vi "Digital_Bridge_3_kart.vi"() -> ()   [LabVIEW 2014] (continued)
        frame Enabled {
        }
      }
      n170 = property class="DAQmx Buffer"(reference=w121, error in=w120, "Input:Buffer Size"=w68) -> (reference out=w80:refnum<k21>, error out=w79:errorcluster)
      n171 = property class="DAQmx Buffer"(reference=w116, error in=w117, "Input:Buffer Size"=w68) -> (reference out=w119:refnum<k21>, error out=w118:errorcluster)
      n172 = property class="DAQmx Buffer"(reference=w115, error in=w114, "Input:Buffer Size"=w68) -> (reference out=w113:refnum<k21>, error out=w112:errorcluster)
      n173 = property class="DAQmx Timing"(reference=w80, error in=w79, "More:Reference Clock:Source"=w58, "RefClk.Rate"=w59) -> (reference out=w78:refnum<k21>, error out=w77:errorcluster)
      n174 = call "Get_Terminal_Name_with_Device_Prefix.vi"("error in (no error)"=w77, "Local Terminal Name"="SyncPulse", "task/channels in"=w78) -> ("error out"=w74:errorcluster, "Terminal Name with Device Prefix"=w60:tag, "task out"=w76:refnum<k21>)  [unwired: 6 in]
      n175 = disable-structure shown="Disabled" {
        disable-tunnel: [w527 _] -> w65
        disable-tunnel: [w526 _] -> w64
        disable-tunnel: w62 -> [w525 _]
        disable-tunnel: w61 -> [w524 _]
        disable-tunnel: w60 -> [w523 _]
        disable-tunnel: w59 -> [w522 _]
        disable-tunnel: w58 -> [w521 _]
        frame Disabled {
          n176 = property class="DAQmx Timing"(reference=w525, error in=w524, "More:Reference Clock:Source"=w521, "RefClk.Rate"=w522, "SyncPulse.Src"=w523) -> (reference out=w527:refnum<k21>, error out=w526:errorcluster)
        }
        frame Enabled {
        }
      }
      n177 = disable-structure shown="Disabled" {
        disable-tunnel: w67 -> [w463 _]
        disable-tunnel: w66 -> [w462 _]
        disable-tunnel: w60 -> [w461 _]
        disable-tunnel: w59 -> [w460 _]
        disable-tunnel: w58 -> [w459 _]
        disable-tunnel: [w458 _] -> w54
        disable-tunnel: [w457 _] -> w53
        frame Disabled {
          n178 = property class="DAQmx Timing" props=["More:Reference Clock:Source", "More:Reference Clock:Rate", "SyncPulse.Src", "SyncPulse.SyncTime"](reference=w463, error in=w462, "More:Reference Clock:Source"=w459, "More:Reference Clock:Rate"=w460, "SyncPulse.Src"=w461) -> (reference out=w458:refnum<k21>, error out=w457:errorcluster)  [unwired: 1 out]
        }
        frame Enabled {
        }
      }
      n179 = property class="DAQmx Timing"(reference=w119, error in=w118, "More:Reference Clock:Source"=w58, "More:Reference Clock:Rate"=w59, "SyncPulse.Src"=w60) -> (reference out=w98:refnum<k21>, error out=w97:errorcluster, "SyncPulse.SyncTime"=w72:dbl)
      n180 = property class="DAQmx Timing" props=["More:Reference Clock:Source", "More:Reference Clock:Rate", "SyncPulse.Src", "SyncPulse.SyncTime"](reference=w113, error in=w112, "More:Reference Clock:Source"=w58, "More:Reference Clock:Rate"=w59, "SyncPulse.Src"=w60) -> (reference out=w96:refnum<k21>, error out=w95:errorcluster)  [unwired: 1 out]
      n181 = property class="DAQmx Timing"(reference=w209, error in=w208, "More:Reference Clock:Source"=w58, "RefClk.Rate"=w59, "SyncPulse.Src"=w60) -> (reference out=w92:refnum<k21>, error out=w91:errorcluster)
      n182 = property class="DAQmx Timing"(reference=w149, error in=w148, "More:Reference Clock:Source"=w58, "RefClk.Rate"=w59, "SyncPulse.Src"=w60) -> (reference out=w82:refnum<k21>, error out=w81:errorcluster)
      n183 = property class="DAQmx Timing"(reference=w147, error in=w146, "More:Reference Clock:Source"=w58, "RefClk.Rate"=w59, "SyncPulse.Src"=w60) -> (reference out=w87:refnum<k21>, error out=w88:errorcluster)
      n184 = property class="DAQmx Timing"(reference=w76, error in=w74, "SyncPulse.MinDelayToStart"=w72) -> (reference out=w75:refnum<k21>, error out=w73:errorcluster)
      n185 = call <vilib>:"Basic Function Generator.vi"("sampling info"=w122, "signal type"=w123) -> ("signal out"=w207:waveform(dbl))  [unwired: 7 in, 2 out]
      n186 = call <vilib>:"Basic Function Generator.vi"("sampling info"=w122, "signal type"=w123, "phase"=0.0) -> ("signal out"=w206:waveform(dbl))  [unwired: 6 in, 2 out]
      n187 = Build Array(w207, w206) -> (w57:waveform(dbl)[])
      n188 = call "Get Full Terminal Name.vi"("error in"=w73, "Local Terminal Name"="ai/StartTrigger", "task/channels in"=w75) -> ("error out"=w93:errorcluster, "Terminal Name with Device Prefix"=w63:tag, "task out"=w94:refnum<k21>)  [unwired: 6 in]
      n189 = flat-sequence {
        tunnel: w98 -> [w581]
        tunnel: w97 -> [w580]
        tunnel: w96 -> [w570]
        tunnel: w95 -> [w569]
        tunnel: [w571] -> w43
        tunnel: [w568] -> w44
        tunnel: [w579] -> w48
        tunnel: [w578] -> w46
        tunnel: w94 -> [w577]
        tunnel: [w577] -> w52
        tunnel: [w576] -> w50
        tunnel: w93 -> [w576]
        tunnel: w63 -> [w567]
        tunnel: w54 -> [w575]
        tunnel: w53 -> [w574]
        tunnel: [w573] -> w40
        tunnel: [w572] -> w38
        frame #0 {
          n190 = disable-structure shown="Disabled" {
            disable-tunnel: w575 -> [w586 _]
            disable-tunnel: w574 -> [w585 _]
            disable-tunnel: [w584 _] -> w573
            disable-tunnel: [w583 _] -> w572
            disable-tunnel: w567 -> [w582 _]
            frame Disabled {
              n191 = call-poly <vilib>:"DAQmx Trigger.vi"("task/channels in"=w586, "source"=w582, "error in"=w585) -> ("task out"=w588:refnum<k21>, "error out"=w587:errorcluster)  [unwired: 11 in]
              n192 = call <vilib>:"DAQmx Start Task.vi"("task/channels in"=w588, "error in"=w587) -> ("task out"=w584:refnum<k21>, "error out"=w583:errorcluster)  [unwired: 12 in]
            }
            frame Enabled {
            }
          }
          n193 = call-poly <vilib>:"DAQmx Trigger.vi"("task/channels in"=w581, "source"=w567, "error in"=w580) -> ("task out"=w579:refnum<k21>, "error out"=w578:errorcluster)  [unwired: 11 in]
          n194 = call-poly <vilib>:"DAQmx Trigger.vi"("task/channels in"=w570, "source"=w567, "error in"=w569) -> ("task out"=w571:refnum<k21>, "error out"=w568:errorcluster)  [unwired: 11 in]
        }
      }
      n195 = disable-structure shown="Disabled" {
        disable-tunnel: w65 -> [w514 _]
        disable-tunnel: w64 -> [w513 _]
        disable-tunnel: w63 -> [w512 _]
        disable-tunnel: w57 -> [w511 _]
        disable-tunnel: [w510 _] -> w56
        disable-tunnel: [w509 _] -> w55
        frame Disabled {
          w518 = 10.0  # timeout (s)
          w517 = FALSE  # auto start
          n196 = call-poly <vilib>:"DAQmx Trigger.vi"("task/channels in"=w514, "source"=w512, "error in"=w513) -> ("task out"=w519:refnum<k21>, "error out"=w520:errorcluster)  [unwired: 11 in]
          n197 = call-poly <vilib>:"DAQmx Write.vi"("task/channels in"=w519, "auto start"=w517, "data"=w511, "timeout"=w518, "error in"=w520) -> ("task out"=w516:refnum<k21>, "error out"=w515:errorcluster)  [unwired: 8 in, 1 out]
          n198 = call <vilib>:"DAQmx Start Task.vi"("task/channels in"=w516, "error in"=w515) -> ("task out"=w510:refnum<k21>, "error out"=w509:errorcluster)  [unwired: 12 in]
        }
        frame Enabled {
        }
      }
      n199 = call-poly <vilib>:"DAQmx Trigger.vi"("task/channels in"=w87, "source"=w63, "error in"=w88) -> ("task out"=w86:refnum<k21>, "error out"=w85:errorcluster)  [unwired: 11 in]
      n200 = call-poly <vilib>:"DAQmx Trigger.vi"("task/channels in"=w92, "source"=w63, "error in"=w91) -> ("task out"=w90:refnum<k21>, "error out"=w89:errorcluster)  [unwired: 11 in]
      n201 = call-poly <vilib>:"DAQmx Trigger.vi"("task/channels in"=w82, "source"=w63, "error in"=w81) -> ("task out"=w83:refnum<k21>, "error out"=w84:errorcluster)  [unwired: 11 in]
      n202 = flat-sequence {
        tunnel: w52 -> [w566]
        tunnel: [w566] -> w51
        tunnel: w50 -> [w565]
        tunnel: [w565] -> w49
        tunnel: w48 -> [w564]
        tunnel: [w564] -> w47
        tunnel: w46 -> [w563]
        tunnel: [w563] -> w45
        tunnel: w44 -> [w562]
        tunnel: w43 -> [w561]
        tunnel: [w560] -> w42
        tunnel: [w559] -> w41
        tunnel: w40 -> [w558]
        tunnel: [w558] -> w39
        tunnel: w38 -> [w557]
        tunnel: [w557] -> w37
        frame #0 {
          n203 = call <vilib>:"DAQmx Start Task.vi"("task/channels in"=w561, "error in"=w562) -> ("task out"=w560:refnum<k21>, "error out"=w559:errorcluster)  [unwired: 12 in]
        }
      }
      n204 = call-poly <vilib>:"DAQmx Write.vi"("task/channels in"=w83, "auto start"=w139, "data"=w57, "timeout"=w138, "error in"=w84) -> ("task out"=w140:refnum<k21>, "error out"=w141:errorcluster)  [unwired: 8 in, 1 out]
      n205 = call-poly <vilib>:"DAQmx Write.vi"("task/channels in"=w86, "auto start"=w144, "data"=w57, "timeout"=w145, "error in"=w85) -> ("task out"=w143:refnum<k21>, "error out"=w142:errorcluster)  [unwired: 8 in, 1 out]
      n206 = call-poly <vilib>:"DAQmx Write.vi"("task/channels in"=w90, "auto start"=w211, "data"=w57, "timeout"=w210, "error in"=w89) -> ("task out"=w214:refnum<k21>, "error out"=w215:errorcluster)  [unwired: 8 in, 1 out]
      n207 = call <vilib>:"DAQmx Start Task.vi"("task/channels in"=w47, "error in"=w45) -> ("task out"=w351:refnum<k21>, "error out"=w350:errorcluster)  [unwired: 12 in]
      n208 = call <vilib>:"DAQmx Start Task.vi"("task/channels in"=w140, "error in"=w141) -> ("task out"=w131:refnum<k21>, "error out"=w130:errorcluster)  [unwired: 12 in]
      n209 = call <vilib>:"DAQmx Start Task.vi"("task/channels in"=w143, "error in"=w142) -> ("task out"=w136:refnum<k21>, "error out"=w137:errorcluster)  [unwired: 12 in]
      n210 = call <vilib>:"DAQmx Start Task.vi"("task/channels in"=w214, "error in"=w215) -> ("task out"=w212:refnum<k21>, "error out"=w213:errorcluster)  [unwired: 12 in]
      n211 = flat-sequence {
        tunnel: w351 -> [w6985]
        tunnel: w350 -> [w6984]
        tunnel: [w6985] -> w347
        tunnel: [w6984] -> w346
        tunnel: [w6983] -> w348
        tunnel: [w6982] -> w349
        tunnel: w51 -> [w6981]
        tunnel: w49 -> [w6980]
        frame #0 {
          n212 = call <vilib>:"DAQmx Start Task.vi"("task/channels in"=w6981, "error in"=w6980) -> ("task out"=w6982:refnum<k21>, "error out"=w6983:errorcluster)  [unwired: 12 in]
        }
      }
      n213 = while {
        stop <- w352 stop-if-true
        n214 = event shown="[3] \"Manuel Setup\": Mouse Down" {
          selector: _ -> [_ _ _ _ _ _]
          dyn-events: _ -> [_ _ _ _ _ _]
          timeout: _ -> [_ _ _ _ _ _]
          event Timeout {
            n215 = event-data() -> ()  [unwired: 1 in, 3 out]
            n216 = flat-sequence {
              frame #0 {
              }
            }
          }
          event "Frekans Listbox": Double Click {
            n217 = event-data() -> ("Row"=w354:i32)  [unwired: 1 in, 8 out]
            n218 = flat-sequence {
              tunnel: w354 -> [w355]
              frame #0 {
                n219 = property on="Frekans Listbox" class="LstBox (strict)"() -> ("Item Symbols"=w359:i32[])  [unwired: 2 in, 2 out]
                n220 = Index Array(array=w359, index=w355) -> (element=w358:i32)
                n221 = Equal?(x=w358, y=10) -> (x = y?=w356:bool)
                n222 = case shown="True" w356 {
                  tunnel: w355 -> [w360 w364]
                  frame False {
                    n223 = property on="Frekans Listbox" class="LstBox (strict)"() -> ("Item Symbols"=w363:i32[])  [unwired: 2 in, 2 out]
                    n224 = Replace Array Subset(array=w363, new element=10 ("new element/subarray"), index=w360) -> (w362:i32[])
                    n225 = property on="Frekans Listbox" class="LstBox (strict)"("Item Symbols"=w362) -> ()  [unwired: 2 in, 2 out]
                  }
                  frame True {
                    n226 = property on="Frekans Listbox" class="LstBox (strict)"() -> ("Item Symbols"=w367:i32[])  [unwired: 2 in, 2 out]
                    n227 = Replace Array Subset(array=w367, new element=1 ("new element/subarray"), index=w364) -> (w366:i32[])
                    n228 = property on="Frekans Listbox" class="LstBox (strict)"("Item Symbols"=w366) -> ()  [unwired: 2 in, 2 out]
                  }
                }
              }
            }
          }
          event "Default Values Listbox": Double Click {
            n229 = event-data() -> ("Row"=w370:i32)  [unwired: 1 in, 8 out]
            n230 = flat-sequence {
              tunnel: w370 -> [w371]
              tunnel: [w372] -> w369
              tunnel: [w371] -> w368
              tunnel: w369 -> [w377]
              tunnel: w368 -> [w376]
              frame #0 {
                n231 = property on="Default Values Listbox" class="LstBox (strict)"() -> ("Item Symbols"=w375:i32[])  [unwired: 2 in, 2 out]
                n232 = Index Array(array=w375, index=w371) -> (element=w374:i32)
                n233 = Equal?(x=w374, y=10) -> (x = y?=w372:bool)
              }
              frame #1 {
                n234 = case shown="True" w377 {
                  tunnel: w376 -> [w378 w402]
                  frame False {
                    n235 = flat-sequence {
                      tunnel: [w382] -> w381
                      tunnel: w378 -> [w382]
                      tunnel: [w382] -> w380
                      tunnel: w381 -> [w390]
                      tunnel: [w387] -> w379
                      tunnel: w380 -> [w387]
                      tunnel: w379 -> [w391]
                      frame #0 {
                      }
                      frame #1 {
                        n236 = local read "F Values Array"() -> (w383:dbl[][])
                        n237 = control-ref of="Default Values Listbox"() -> (w384:refnum<vi>)
                        n238 = property on="Default Values Listbox" class="LstBox (strict)"() -> ("Item Names"=w389:string[])  [unwired: 2 in, 2 out]
                        n239 = Fract/Exp String To Number(string=w389) -> (number=w388:dbl[])  [unwired: 3 in, 1 out]
                        n240 = Index Array(array=w388, index=w390) -> (element=w386:dbl)
                        n241 = call "delete_values.vi"("F values array"=w383, "Frekans"=w386, "LstBox Refnum"=w384) -> ("Output F values array"=w385:dbl[][])  [unwired: 8 in]
                        n242 = local write "F Values Array"(w385) -> ()
                      }
                      frame #2 {
                        n243 = property on="Default Values Listbox" class="LstBox (strict)"() -> ("Item Symbols"=w394:i32[])  [unwired: 2 in, 2 out]
                        n244 = Replace Array Subset(array=w394, new element=10 ("new element/subarray"), index=w391) -> (w393:i32[])
                        n245 = property on="Default Values Listbox" class="LstBox (strict)"("Item Symbols"=w393) -> ()  [unwired: 2 in, 2 out]
                      }
                    }
                  }
                  frame True {
                    n246 = flat-sequence {
                      tunnel: [w405] -> w403
                      tunnel: w402 -> [w405]
                      tunnel: [w406] -> w401
                      tunnel: [w405] -> w400
                      tunnel: w403 -> [w408]
                      tunnel: w401 -> [w415]
                      tunnel: [w412] -> w398
                      tunnel: w400 -> [w412]
                      tunnel: [w408] -> w396
                      tunnel: w398 -> [w420]
                      tunnel: [w420] -> w397
                      tunnel: w396 -> [w419]
                      tunnel: [w419] -> w395
                      tunnel: w397 -> [w423]
                      tunnel: [w423] -> w399
                      tunnel: w395 -> [w421]
                      tunnel: w399 -> [w424]
                      frame #0 {
                        n247 = local read "Sheet name"() -> (w404:string)
                        n248 = call "Excel Get Data Specified Field.vi"("SheetName"=w404) -> ("data"=w407:string[][])  [unwired: 4 in, 2 out]
                        n249 = Fract/Exp String To Number(string=w407) -> (number=w406:dbl[][])  [unwired: 3 in, 1 out]
                      }
                      frame #1 {
                        n250 = local read "F Values Array"() -> (w409:dbl[][])
                        n251 = control-ref of="Default Values Listbox"() -> (w410:refnum<vi>)
                        n252 = Reshape Array(w415, 51 ("dimension size")) -> (w413:dbl[])
                        n253 = property on="Default Values Listbox" class="LstBox (strict)"() -> ("Item Names"=w418:string[])  [unwired: 2 in, 2 out]
                        n254 = Fract/Exp String To Number(string=w418) -> (number=w417:dbl[])  [unwired: 3 in, 1 out]
                        n255 = Index Array(array=w417, index=w408) -> (element=w416:dbl)
                        n256 = call "add_values.vi"("F values array"=w409, "Values"=w413, "Frekans"=w416, "LstBox Refnum"=w410) -> ("Output F values array"=w411:dbl[][])  [unwired: 7 in]
                        n257 = local write "F Values Array"(w411) -> ()
                      }
                      frame #2 {
                      }
                      frame #3 {
                        n258 = local read "F Values Array"() -> (w422:dbl[][])
                        n259 = call "rlc warning.vi"("frekans index"=w421, "F values array"=w422) -> ()  [unwired: 10 in]
                      }
                      frame #4 {
                        n260 = property on="Default Values Listbox" class="LstBox (strict)"() -> ("Item Symbols"=w427:i32[])  [unwired: 2 in, 2 out]
                        n261 = Replace Array Subset(array=w427, new element=1 ("new element/subarray"), index=w424) -> (w426:i32[])
                        n262 = property on="Default Values Listbox" class="LstBox (strict)"("Item Symbols"=w426) -> ()  [unwired: 2 in, 2 out]
                      }
                    }
                  }
                }
              }
            }
          }
          event "Manuel Setup": Mouse Down {
            n263 = event-data() -> ()  [unwired: 1 in, 8 out]
            n264 = local read "Sheet name"() -> (w431:string)
            n265 = call "Excel Get Data Specified Field.vi"("SheetName"=w431) -> ("data"=w432:string[][])  [unwired: 4 in, 2 out]
            n266 = Fract/Exp String To Number(string=w432) -> (number=w433:dbl[][])  [unwired: 3 in, 1 out]
            n267 = Reshape Array(w433, 51 ("dimension size")) -> (w428:dbl[])
            n268 = for {
              N: 51 -> [_]
              tunnel: w428 -> [w435]
              i -> [w436]
              n269 = Index Array(array=w435, index=w436) -> (element=w434:dbl)
              n270 = case shown="0, Default" w436 {
                tunnel: w434 -> [w437 w438 _ _ _ _ _ _ _ w439 w440 w441 w442 w443 _ _ _ _ _ w444 w445 w446 w447 w448 _ _ _ _ _ _ _ _ _ _ _ _ _ _ _ _ _ _ _ _ _ _ _ _ _ _ _]
                frame 0, Default {
                  n271 = global write "DB_Global_4_kart-Test.vi" "Frequency"(w437) -> ()
                }
                frame 1 {
                  n272 = global write "DB_Global_4_kart-Test.vi" "amplitude 1/0"(w438) -> ()
                }
                frame 2 {
                }
                frame 3 {
                }
                frame 4 {
                }
                frame 5 {
                }
                frame 6 {
                }
                frame 7 {
                }
                frame 8 {
                }
                frame 9 {
                  n273 = global write "DB_Global_4_kart-Test.vi" "amplitude 2/0"(w439) -> ()
                }
                frame 10 {
                  n274 = global write "DB_Global_4_kart-Test.vi" "amplitude 3/0"(w440) -> ()
                }
                frame 11 {
                  n275 = global write "DB_Global_4_kart-Test.vi" "amplitude 3/1"(w441) -> ()
                }
                frame 12 {
                  n276 = global write "DB_Global_4_kart-Test.vi" "amplitude 1/1"(w442) -> ()
                }
                frame 13 {
                  n277 = global write "DB_Global_4_kart-Test.vi" "amplitude 2/1"(w443) -> ()
                }
                frame 14 {
                }
                frame 15 {
                }
                frame 16 {
                }
                frame 17 {
                }
                frame 18 {
                }
                frame 19 {
                  n278 = global write "DB_Global_4_kart-Test.vi" "phase 2/ 0"(w444) -> ()
                }
                frame 20 {
                  n279 = global write "DB_Global_4_kart-Test.vi" "phase 3/0"(w445) -> ()
                }
                frame 21 {
                  n280 = global write "DB_Global_4_kart-Test.vi" "phase 3/1"(w446) -> ()
                }
                frame 22 {
                  n281 = global write "DB_Global_4_kart-Test.vi" "phase 1/1"(w447) -> ()
                }
                frame 23 {
                  n282 = global write "DB_Global_4_kart-Test.vi" "phase 2/1"(w448) -> ()
                }
                frame 24 {
                }
                frame 25 {
                }
                frame 26 {
                }
                frame 27 {
                }
                frame 28 {
                }
                frame 29 {
                }
                frame 30 {
                }
                frame 31 {
                }
                frame 32 {
                }
                frame 33 {
                }
                frame 34 {
                }
                frame 35 {
                }
                frame 36 {
                }
                frame 37 {
                }
                frame 38 {
                }
                frame 39 {
                }
                frame 40 {
                }
                frame 41 {
                }
                frame 42 {
                }
                frame 43 {
                }
                frame 44 {
                }
                frame 45 {
                }
                frame 46 {
                }
                frame 47 {
                }
                frame 48 {
                }
                frame 49 {
                }
                frame 50 {
                }
              }
            }
          }
          event "Multicolumn Listbox": Mouse Down {
            n283 = event-data() -> ("Coords"=w450:T8)  [unwired: 1 in, 7 out]
            n284 = invoke on="Multicolumn Listbox" class="MCListbox (strict)" method="Point To Row Column"("Point"=w450) -> ("CellPosition"=w449:T9)  [unwired: 6 in, 6 out]
            n285 = property on="Multicolumn Listbox" class="MCListbox (strict)"("EditPos"=w449) -> ()  [unwired: 2 in, 2 out]
          }
          event "Manuel Input": Mouse Down {
            n286 = event-data() -> ()  [unwired: 1 in, 8 out]
            n287 = call <vilib>:"System Exec.vi"("command line"="cmd /c start \"\" \"D:\\Projeler\\Digital Bridge\\Digital_Bridge_3_kart\\Manuel.vi\"") -> ()  [unwired: 7 in, 4 out]
          }
        }
        n288 = Wait (ms)(milliseconds to wait=u32 50) -> ()  [unwired: 1 out]
        n289 = local read "stop listbox"() -> (w352:bool)
      }
      n290 = while {
        shift-right: [w636] -> w344
        shift-left: w348 -> [w636]
        shift-right: [w634] -> w340
        shift-left: w346 -> [w634]
        shift-right: [w637] -> w345
        shift-left: w349 -> [w637]
        shift-right: [w635] -> w341
        shift-left: w347 -> [w635]
        shift-right: [w633] -> w332
        shift-left: w42 -> [w633]
        shift-right: [w632] -> w331
        shift-left: w41 -> [w632]
        shift-right: [w640] -> w203
        shift-left: w213 -> [w655]
        shift-right: [w654] -> w204
        shift-left: w212 -> [w653]
        shift-right: [w639] -> w133
        shift-left: w137 -> [w649]
        shift-right: [w650] -> w132
        shift-left: w136 -> [w651]
        shift-right: [w645] -> w127
        shift-left: w131 -> [w646]
        shift-right: [w638] -> w126
        shift-left: w130 -> [w644]
        shift-right: [w627] -> w36
        shift-left: w56 -> [w629]
        shift-right: [w626] -> w35
        shift-left: w55 -> [w628]
        shift-right: [w625] -> w33
        shift-left: w39 -> [w625]
        shift-right: [w624] -> w32
        shift-left: w37 -> [w624]
        stop <- w619 stop-if-true
        w652 = FALSE  # auto start
        # "Bu bölümde, input değerleri sürekli güncellenir. \n\nGüncel tutulan bu input değerleri, daha sonra Excel dosyasına aktarılacak ölçüm sonuçlarıdır."
        # "Bu bölümde, denge koşullarını değiştirmek istediğimiz listbox’un kodları bulunur. \n\nYani, kullanıcının listbox üzerinden seçtiği denge koşullarına göre programın davranışını belirleyen işlemler burada gerçekleştirilir."
        # "Bu bölüm, eğer giriş değeri 8V’dan büyükse ya da ölçüm sayısı (meas number) belirlenen sınırı aşarsa aktif olur. \n\nBu durumda, ilgili frekans için “dengelenemedi” mesajı atanır. \n\nAncak program, sonraki turlarda bu frekans için tekrar dengeleme denemelerine devam eder."
        # "Bu bölüm, ya tüm dengeler başarıyla sağlandığında ya da bir hata (error) durumunda aktif olur. \n\nEğer ölçüm yapılan frekansta dengeleme tamamlanmışsa, program mevcut frekanstan doğrudan sonraki frekansa geçiş yapar. \n\nHata oluşmuşsa da yine diğer frekansa geçiş için gerekli hazırlıklar burada yapılır. \n\nKısaca, bu case bir frekans tamamlandığında diğerine geçiş için ön hazırlıkların yapıldığı yerdir."
        # "Bu bölüm, program ilk kez başlatıldığında yapılması gereken başlangıç işlemlerini içerir. \n\nÖrneğin; faz için 2 boyutlu dizilerin (2D array) oluşturulması, programdaki birçok değişkenin ve değerlerin sıfırlanması gibi temel ayarlamalar burada yapılır. \n\nBu sayede program, temiz ve hazır bir durumda çalışmaya başlar."
        # "BASLAT: \n\nBu bölüm, kullanıcı ana programda gerekli tüm ayarları yaptıktan sonra \"Başlat\" düğmesine bastığında çalışır. Programın başlamasından önce bazı kontroller yapılır. Örneğin, kullanıcı geçerli bir frekans seçmiş mi, ölçüm ve set değerleri 100’ün üzerinde mi, gerekli global giriş değerleri girilmiş mi gibi durumlar kontrol edilir. Bu kontroller sayesinde eksik veya hatalı girişler varsa kullanıcıya uyarı verilir. \n\nAynı zamanda bu bölüm, programın düzgün çalışabilmesi için gerekli olan temel verilerin oluşturulduğu alandır. Control Hz, frekanslar, ekstra varsayılan değerler, denge fazlarını içeren diziler ve bazı cluster yapıları burada tanımlanır. Eğer kullanıcı Excel’den veri aldıysa, bu veriler de burada işlenerek F values dizisine aktarılır. Kısacası, programın başlaması için gerekli olan tüm başlangıç ayarları ve veri hazırlıkları bu case içinde yapılır."
        # "Dev3"
        # "Dev2"
        # "Dev1"
        # "Slot2"
        n291 = flat-sequence {
          tunnel: [w4175] -> w601
          tunnel: [w4174] -> w600
          tunnel: [w4173] -> w599
          tunnel: [w4179] -> w621
          tunnel: w601 -> [w4180]
          tunnel: w600 -> [w4181]
          tunnel: w599 -> [w4178]
          tunnel: [w4245] -> w643
          tunnel: [w4237] -> w642
          tunnel: [w4234] -> w641
          tunnel: [w4193] -> w630
          tunnel: w621 -> [w4189]
          frame #0 {
            n292 = local read "frekans index"() -> (w4176:dbl)
            n293 = local read "Frekanslar"() -> (w4177:dbl[])
            n294 = global read "DB_Global_4_kart-Test.vi" "Manuel Kullan"() -> (w4174:bool)
            n295 = global read "DB_Global_4_kart-Test.vi" "Frequency"() -> (w4175:dbl)
            n296 = Index Array(array=w4177, index=w4176) -> (element=w4173:dbl)
          }
          frame #1 {
            n297 = case shown="False" w4181 {
              tunnel: [w4183 w4188] -> w4179
              tunnel: w4180 -> [_ w4188]
              tunnel: w4178 -> [w4182 _]
              frame False {
                n298 = Less Or Equal?(x=w4182, y=0.0) -> (x <= y?=w4184:bool)
                n299 = case shown="True" w4184 {
                  tunnel: [w4186 1000.0] -> w4183
                  tunnel: w4182 -> [w4186 _]
                  frame False {
                  }
                  frame True {
                  }
                }
              }
              frame True {
              }
            }
          }
          frame #2 {
            w4192 = 0.0 ("Offset")
            # "Yedek Kart ao1"
            # "Yedek Kart ao0"
            # "1R Voltajı"
            # "Kelvin Voltajı"
            # "Wagner Voltajı"
            # "10R Voltajı"
            # "Ana Denge Voltajı"
            # "Besleme Voltajı"
            n300 = global read "DB_Global_4_kart-Test.vi" "amplitude 1/0"() -> (w4214:dbl)
            n301 = global read "DB_Global_4_kart-Test.vi" "phase 1/ 0"() -> (w4212:dbl)
            n302 = global read "DB_Global_4_kart-Test.vi" "amplitude 1/1"() -> (w4213:dbl)
            n303 = global read "DB_Global_4_kart-Test.vi" "phase 1/1"() -> (w4218:dbl)
            n304 = global read "DB_Global_4_kart-Test.vi" "amplitude 2/0"() -> (w4232:dbl)
            n305 = global read "DB_Global_4_kart-Test.vi" "phase 2/ 0"() -> (w4233:dbl)
            n306 = global read "DB_Global_4_kart-Test.vi" "amplitude 2/1"() -> (w4211:dbl)
            n307 = global read "DB_Global_4_kart-Test.vi" "phase 2/1"() -> (w4210:dbl)
            n308 = global read "DB_Global_4_kart-Test.vi" "amplitude 3/0"() -> (w4228:dbl)
            n309 = global read "DB_Global_4_kart-Test.vi" "phase 3/0"() -> (w4227:dbl)
            n310 = global read "DB_Global_4_kart-Test.vi" "amplitude 3/1"() -> (w4223:dbl)
            n311 = global read "DB_Global_4_kart-Test.vi" "phase 3/1"() -> (w4222:dbl)
            n312 = global read "DB_Global_4_kart-Test.vi" "amplitude 5/0"() -> (w4199:dbl)
            n313 = global read "DB_Global_4_kart-Test.vi" "phase 5/0"() -> (w4198:dbl)
            n314 = global read "DB_Global_4_kart-Test.vi" "amplitude 5/1"() -> (w4202:dbl)
            n315 = global read "DB_Global_4_kart-Test.vi" "phase 5/1"() -> (w4203:dbl)
            n316 = global write "DB_Global_4_kart-Test.vi" "Frequency"(w4189) -> ()
            n317 = Re/Im To Polar(2:w4203, 3:w4202) -> (0:w4205:dbl, 1:w4204:dbl)
            n318 = Re/Im To Polar(2:w4210, 3:w4211) -> (0:w4208:dbl, 1:w4209:dbl)
            n319 = Re/Im To Polar(2:w4198, 3:w4199) -> (0:w4200:dbl, 1:w4191:dbl)
            n320 = Re/Im To Polar(2:w4227, 3:w4228) -> (0:w4225:dbl, 1:w4226:dbl)
            n321 = Re/Im To Polar(2:w4222, 3:w4223) -> (0:w4220:dbl, 1:w4221:dbl)
            n322 = Re/Im To Polar(2:w4218, 3:w4213) -> (0:w4216:dbl, 1:w4217:dbl)
            n323 = expression code="(x/pi)*180.0" ("radians to degrees")(w4205) -> (w4206:dbl)
            n324 = expression code="(x/pi)*180.0" ("radians to degrees")(w4208) -> (w4207:dbl)
            n325 = expression code="(x/pi)*180.0" ("radians to degrees")(w4200) -> (w4201:dbl)
            n326 = Re/Im To Polar(2:w4233, 3:w4232) -> (0:w4230:dbl, 1:w4231:dbl)
            n327 = expression code="(x/pi)*180.0" "radians to degrees"(w4220) -> (w4219:dbl)
            n328 = expression code="(x/pi)*180.0" ("radians to degrees")(w4225) -> (w4224:dbl)
            n329 = expression code="(x/pi)*180.0" ("radians to degrees")(w4216) -> (w4215:dbl)
            n330 = expression code="(x/pi)*180.0" ("radians to degrees")(w4230) -> (w4229:dbl)
            n331 = call "Simulate Signal2"("Offset"=w4192, "Reset Signal"=TRUE, "Frequency"=w4189, "Amplitude"=w4217, "Phase"=w4215) -> ("Sine"=w4246:dynamicdata)  [unwired: 9 in, 1 out]
            n332 = call "Simulate Signal8"("Offset"="Yedek Kart offset", "Reset Signal"=TRUE, "Frequency"=w4189, "Amplitude"=w4204, "Phase"=w4206) -> ("Sine"=w4196:dynamicdata)  [unwired: 9 in, 1 out]
            n333 = call "Simulate Signal"("Offset"=w4192, "Reset Signal"=TRUE, "Frequency"=w4189, "Amplitude"=w4214, "Phase"=w4212) -> ("Sine"=w4247:dynamicdata)  [unwired: 9 in, 1 out]
            n334 = call "Simulate Signal7"("Offset"="Yedek Kart offset", "Reset Signal"=TRUE, "Frequency"=w4189, "Amplitude"=w4191, "Phase"=w4201) -> ("Sine"=w4197:dynamicdata)  [unwired: 9 in, 1 out]
            n335 = call "Simulate Signal5"("Offset"=w4192, "Reset Signal"=TRUE, "Frequency"=w4189, "Amplitude"=w4226, "Phase"=w4224) -> ("Sine"=w4235:dynamicdata)  [unwired: 9 in, 1 out]
            n336 = call "Simulate Signal6"("Offset"=w4192, "Reset Signal"=TRUE, "Frequency"=w4189, "Amplitude"=w4221, "Phase"=w4219) -> ("Sine"=w4236:dynamicdata)  [unwired: 9 in, 1 out]
            n337 = call "Simulate Signal3"("Offset"=w4192, "Reset Signal"=TRUE, "Frequency"=w4189, "Amplitude"=w4231, "Phase"=w4229) -> ("Sine"=w4238:dynamicdata)  [unwired: 9 in, 1 out]
            n338 = call "Simulate Signal4"("Offset"=w4192, "Reset Signal"=TRUE, "Frequency"=w4189, "Amplitude"=w4209, "Phase"=w4207) -> ("Sine"=w4239:dynamicdata)  [unwired: 9 in, 1 out]
            n339 = Build Array(w4197, w4196) -> (w4193:dynamicdata[])
            n340 = Build Array(w4235, w4236) -> (w4234:dynamicdata[])
            n341 = Build Array(w4247, w4246) -> (w4245:dynamicdata[])
            n342 = Build Array(w4238, w4239) -> (w4237:dynamicdata[])
          }
        }
        n343 = case shown="True" "BASLAT" {
          tunnel: "Fazları ve ilk denge koşulu dengelemek için gerekli range ve input değerleri verdiniz mi?\n[Bu kısım önemli çünkü ilk range ve input değerleri fazların doğru girilmesi için önem arz ediyor.]" -> [_ w1132]
          frame False {
          }
          frame True {
            n344 = local read "start time"() -> (w1134:string)
            n345 = String Length(string=w1134) -> (length=w1135:i32)
            n346 = Equal?(x=w1135, y=0) -> (x = y?=w1133:bool)
            n347 = case shown="True" w1133 {
              tunnel: [TRUE ("T button?") w1142] -> w1137
              tunnel: w1132 -> [_ w1139]
              frame False {
              }
              frame True {
                n348 = Two Button Dialog(message=w1139, 1:"Ayarla", 2:"Evet") -> (T button?=w1142:bool)
              }
            }
            n349 = case shown="True" w1137 {
              frame False {
                n350 = One Button Dialog(message="Değerleri girdikten sonra ana programı tekrardan başlatmayı unutmayın", button name ("OK")="Tamam") -> (true=w1143:bool)
                n351 = case shown="True" w1143 {
                  frame False {
                  }
                  frame True {
                    n352 = local write "BASLAT"(FALSE ("BASLAT")) -> ()
                    n353 = local write "Stop"(TRUE ("BASLAT")) -> ()
                    n354 = call <vilib>:"System Exec.vi"("command line"="cmd /c start \"\" \"D:\\Projeler\\Digital Bridge\\Digital_Bridge_3_kart\\First_input_values.vi\"") -> ()  [unwired: 7 in, 4 out]
                  }
                }
              }
              frame True {
                n355 = local read "start time"() -> (w1153:string)
                n356 = String Length(string=w1153) -> (length=w1152:i32)
                n357 = Equal?(x=w1152, y=0) -> (x = y?=w1151:bool)
                n358 = case shown="True" w1151 {
                  tunnel: [TRUE w1155] -> w1150
                  frame False {
                  }
                  frame True {
                    n359 = flat-sequence {
                      tunnel: [w1156] -> w1155
                      frame #0 {
                        n360 = control-ref of="Frekans Listbox"() -> (w1160:refnum<vi>)
                        n361 = case shown="0, Default" "Direnc 1 - Direnc 2" {
                          frame 0, Default {
                            n362 = local write "Direnc 1 [ohm]"(1000000.0 ("Direnc 1 [ohm]")) -> ()
                            n363 = local write "Direnc 2 [ohm]"(100000.0 ("Direnc 1 [ohm]")) -> ()
                          }
                          frame 1 {
                            n364 = local write "Direnc 1 [ohm]"(100000.0 ("Direnc 1 [ohm]")) -> ()
                            n365 = local write "Direnc 2 [ohm]"(10000.0 ("Direnc 1 [ohm]")) -> ()
                          }
                          frame 2 {
                            n366 = local write "Direnc 1 [ohm]"(10000.0 ("Direnc 1 [ohm]")) -> ()
                            n367 = local write "Direnc 2 [ohm]"(1000.0 ("Direnc 1 [ohm]")) -> ()
                          }
                          frame 3 {
                            n368 = local write "Direnc 1 [ohm]"(1000.0 ("Direnc 1 [ohm]")) -> ()
                            n369 = local write "Direnc 2 [ohm]"(100.0 ("Direnc 1 [ohm]")) -> ()
                          }
                          frame 4 {
                            n370 = local write "Direnc 1 [ohm]"(100.0 ("Direnc 1 [ohm]")) -> ()
                            n371 = local write "Direnc 2 [ohm]"(10.0 ("Direnc 1 [ohm]")) -> ()
                          }
                          frame 5 {
                            n372 = local write "Direnc 1 [ohm]"(10.0 ("Direnc 1 [ohm]")) -> ()
                            n373 = local write "Direnc 2 [ohm]"(1.0 ("Direnc 1 [ohm]")) -> ()
                          }
                          frame 6 {
                            n374 = local write "Direnc 1 [ohm]"(1000000.0 ("Direnc 1 [ohm]")) -> ()
                            n375 = local write "Direnc 2 [ohm]"(1000000.0 ("Direnc 1 [ohm]")) -> ()
                          }
                          frame 7 {
                            n376 = local write "Direnc 1 [ohm]"(100000.0 ("Direnc 1 [ohm]")) -> ()
                            n377 = local write "Direnc 2 [ohm]"(100000.0 ("Direnc 1 [ohm]")) -> ()
                          }
                          frame 8 {
                            n378 = local write "Direnc 1 [ohm]"(10000.0 ("Direnc 1 [ohm]")) -> ()
                            n379 = local write "Direnc 2 [ohm]"(10000.0 ("Direnc 1 [ohm]")) -> ()
                          }
                          frame 9 {
                            n380 = local write "Direnc 1 [ohm]"(1000.0 ("Direnc 1 [ohm]")) -> ()
                            n381 = local write "Direnc 2 [ohm]"(1000.0 ("Direnc 1 [ohm]")) -> ()
                          }
                          frame 10 {
                            n382 = local write "Direnc 1 [ohm]"(100.0 ("Direnc 1 [ohm]")) -> ()
                            n383 = local write "Direnc 2 [ohm]"(100.0 ("Direnc 1 [ohm]")) -> ()
                          }
                          frame 11 {
                            n384 = local write "Direnc 1 [ohm]"(10.0 ("Direnc 1 [ohm]")) -> ()
                            n385 = local write "Direnc 2 [ohm]"(10.0 ("Direnc 1 [ohm]")) -> ()
                          }
                          frame 12 {
                            n386 = local write "Direnc 1 [ohm]"(1.0 ("Direnc 1 [ohm]")) -> ()
                            n387 = local write "Direnc 2 [ohm]"(1.0 ("Direnc 1 [ohm]")) -> ()
                          }
                          frame 13 {
                            n388 = local write "Direnc 1 [ohm]"(1e-06 ("Direnc 1 [ohm]")) -> ()
                            n389 = local write "Direnc 2 [ohm]"(1e-07 ("Direnc 1 [ohm]")) -> ()
                          }
                          frame 14 {
                            n390 = local write "Direnc 1 [ohm]"(1e-07 ("Direnc 1 [ohm]")) -> ()
                            n391 = local write "Direnc 2 [ohm]"(1e-08 ("Direnc 1 [ohm]")) -> ()
                          }
                          frame 15 {
                            n392 = local write "Direnc 1 [ohm]"(1e-08 ("Direnc 1 [ohm]")) -> ()
                            n393 = local write "Direnc 2 [ohm]"(1e-09 ("Direnc 1 [ohm]")) -> ()
                          }
                          frame 16 {
                            n394 = local write "Direnc 1 [ohm]"(1e-09 ("Direnc 1 [ohm]")) -> ()
                            n395 = local write "Direnc 2 [ohm]"(1e-10 ("Direnc 1 [ohm]")) -> ()
                          }
                          frame 17 {
                            n396 = local write "Direnc 1 [ohm]"(1e-10 ("Direnc 1 [ohm]")) -> ()
                            n397 = local write "Direnc 2 [ohm]"(1e-11 ("Direnc 1 [ohm]")) -> ()
                          }
                          frame 18 {
                            n398 = local write "Direnc 1 [ohm]"(1e-11 ("Direnc 1 [ohm]")) -> ()
                            n399 = local write "Direnc 2 [ohm]"(1e-12 ("Direnc 1 [ohm]")) -> ()
                          }
                          frame 19 {
                            n400 = local write "Direnc 1 [ohm]"(1e-06 ("Direnc 1 [ohm]")) -> ()
                            n401 = local write "Direnc 2 [ohm]"(1e-06 ("Direnc 1 [ohm]")) -> ()
                          }
                          frame 20 {
                            n402 = local write "Direnc 1 [ohm]"(1e-07 ("Direnc 1 [ohm]")) -> ()
                            n403 = local write "Direnc 2 [ohm]"(1e-07 ("Direnc 1 [ohm]")) -> ()
                          }
                          frame 21 {
                            n404 = local write "Direnc 1 [ohm]"(1e-08 ("Direnc 1 [ohm]")) -> ()
                            n405 = local write "Direnc 2 [ohm]"(1e-08 ("Direnc 1 [ohm]")) -> ()
                          }
                          frame 22 {
                            n406 = local write "Direnc 1 [ohm]"(1e-09 ("Direnc 1 [ohm]")) -> ()
                            n407 = local write "Direnc 2 [ohm]"(1e-09 ("Direnc 1 [ohm]")) -> ()
                          }
                          frame 23 {
                            n408 = local write "Direnc 1 [ohm]"(1e-10 ("Direnc 1 [ohm]")) -> ()
                            n409 = local write "Direnc 2 [ohm]"(1e-10 ("Direnc 1 [ohm]")) -> ()
                          }
                          frame 24 {
                            n410 = local write "Direnc 1 [ohm]"(1e-11 ("Direnc 1 [ohm]")) -> ()
                            n411 = local write "Direnc 2 [ohm]"(1e-11 ("Direnc 1 [ohm]")) -> ()
                          }
                          frame 25 {
                            n412 = local write "Direnc 1 [ohm]"(1e-12 ("Direnc 1 [ohm]")) -> ()
                            n413 = local write "Direnc 2 [ohm]"(1e-12 ("Direnc 1 [ohm]")) -> ()
                          }
                        }
                        n414 = call "set_frekans_array.vi"("LstBox Refnum"=w1160) -> ("Array"=w1161:dbl[])  [unwired: 10 in]
                        n415 = Array Size(array=w1161) -> (size(s)=w1162:i32)
                        n416 = Greater?(x=w1162, y=0) -> (0:w1157:bool)
                        n417 = case shown="True" w1157 {
                          tunnel: [FALSE w1227] -> w1156
                          frame False {
                            n418 = One Button Dialog(message="En az 1 tane frekans seçmelisiniz!", button name ("OK")="TAMAM") -> (true=w1218:bool)
                            n419 = case shown="True" w1218 {
                              frame False {
                              }
                              frame True {
                              }
                            }
                          }
                          frame True {
                            n420 = Greater?(x="olcum", y=u16 0) -> (0:w1229:bool)
                            n421 = Less?(x="olcum", y=u16 101) -> (x < y?=w1230:bool)
                            n422 = And(x=w1230, y=w1229) -> (x .and. y?=w1220:bool)
                            n423 = Greater?(x="set", y=u16 0) -> (0:w1226:bool)
                            n424 = Less?(x="set", y=u16 101) -> (x < y?=w1225:bool)
                            n425 = And(x=w1225, y=w1226) -> (x .and. y?=w1219:bool)
                            n426 = And(x=w1220, y=w1219) -> (x .and. y?=w1222:bool)
                            n427 = case shown="False" w1222 {
                              tunnel: [FALSE TRUE] -> w1227
                              frame False {
                                n428 = One Button Dialog(message="n1 ve n2 en az 1\n en fazla 100 olmalı", button name ("OK")="TAMAM") -> (true=w1236:bool)
                                n429 = case shown="True" w1236 {
                                frame False {
                                }
                                frame True {
                                }
                                }
                              }
                              frame True {
                              }
                            }
                          }
                        }
                      }
                    }
                  }
                }
                n430 = case shown="True" w1150 {
                  tunnel: w1151 -> [_ w1239]
                  frame False {
                    n431 = local write "BASLAT"(FALSE ("BASLAT")) -> ()
                  }
                  frame True {
                    n432 = flat-sequence {
                      tunnel: w1239 -> [w1240]
                      frame #0 {
                        n433 = case shown="True" w1240 {
                          frame False {
                          }
                          frame True {
                            n434 = flat-sequence {
                              frame #0 {
                                n435 = control-ref of="Frekans Listbox"() -> (w1242:refnum<vi>)
                                n436 = call "set_frekans_array.vi"("LstBox Refnum"=w1242) -> ("Array"=w1241:dbl[])  [unwired: 10 in]
                                n437 = local write "Frekanslar"(w1241) -> ()
                              }
                              frame #1 {
                                n438 = local read "Frekanslar"() -> (w1244:dbl[])
                                n439 = Build Array(w1244) -> (w1243:dbl[][])
                                n440 = local write "control hz array"(w1243) -> ()
                                "frekans index" <- 0.0 ("frekans index")
                              }
                              frame #2 {
                                n441 = for {
                                N: 3 -> [_]
                                i -> [w1249]
                                n442 = Increment(x=w1249) -> (x+1=w1248:i32)
                                n443 = local read "control hz array"() -> (w1251:dbl[][])
                                n444 = Insert Into Array(array=w1251, index (row)=w1248, new element=dbl[] [] ("new element/subarray")) -> (w1252:dbl[][])  [unwired: 1 in]
                                n445 = local write "control hz array"(w1252) -> ()
                                n446 = Wait (ms)(milliseconds to wait=u32 50) -> ()  [unwired: 1 out]
                                }
                              }
                              frame #3 {
                                n447 = local read "Frekanslar"() -> (w1254:dbl[])
                                n448 = Array Size(array=w1254) -> (size(s)=w1253:i32)
                                n449 = call "default cluster.vi"("size"=w1253) -> ("Array"=→"default values":T10)  [unwired: 10 in]
                              }
                              frame #4 {
                                n450 = local read "extra default values"() -> (w1257:dbl[][])
                                n451 = local read "olcum"() -> (w1264:u16)
                                n452 = local read "set"() -> (w1263:u16)
                                n453 = local read "Frekanslar"() -> (w1260:dbl[])
                                n454 = Multiply(x=w1264, y=w1263) -> (x*y=w1262:u16)
                                n455 = Multiply(x=u16 2, y=w1262) -> (x*y=w1261:u16)
                                n456 = Array Size(array=w1260) -> (size(s)=w1259:i32)
                                n457 = call "default zero array.vi"("Array"=dbl[] [], "frekans size"=w1259, "size"=w1261, "control hz array"=w1257) -> ("output array"=w1265:dbl[][])  [unwired: 7 in]
                                n458 = local write "extra default values"(w1265) -> ()
                              }
                            }
                          }
                        }
                      }
                      frame #1 {
                        n459 = Wait (ms)(milliseconds to wait=u32 500) -> ()  [unwired: 1 out]
                      }
                      frame #2 {
                        n460 = flat-sequence {
                          frame #0 {
                            n461 = local read "frekans index"() -> (w1316:dbl)
                            n462 = local read "Frekanslar"() -> (w1315:dbl[])
                            n463 = Index Array(array=w1315, index=w1316) -> (element=w1314:dbl)
                            n464 = property on="Default Values Listbox" class="LstBox (strict)"() -> ("Item Names"=w1321:string[])  [unwired: 2 in, 2 out]
                            n465 = Fract/Exp String To Number(string=w1321) -> (number=w1320:dbl[])  [unwired: 3 in, 1 out]
                            n466 = Search 1D Array(1D array=w1320, element=w1314, start index (0)=0) -> (index of element=w1318:i32)
                            n467 = property on="Default Values Listbox" class="LstBox (strict)"() -> ("Item Symbols"=w1319:i32[])  [unwired: 2 in, 2 out]
                            n468 = Index Array(array=w1319, index=w1318) -> (element=w1313:i32)
                            "1 or 10" <- w1313
                            n469 = case shown="1" w1313 {
                              frame 10, Default {
                              }
                              frame 1 {
                                n470 = local read "AD F/P Array"() -> (w1330:dbl[][])
                                n471 = local read "Wagner F/P Array"() -> (w1328:dbl[][])
                                n472 = local read "10R F/P Array"() -> (w1329:dbl[][])
                                n473 = local read "Direnc 1 - Direnc 2"() -> (w1327:u32)
                                n474 = local read "Frekanslar"() -> (w1334:dbl[])
                                n475 = local read "frekans index"() -> (w1333:dbl)
                                n476 = local read "1R F/P Array"() -> (w1331:dbl[][])
                                n477 = local read "Kelvin F/P Array"() -> (w1332:dbl[][])
                                n478 = local read "F Values Array"() -> (w1335:dbl[][])
                                n479 = control-ref of="Default Values Listbox"() -> (w1336:refnum<vi>)
                                n480 = call "set_fp_array.vi"("LstBox Refnum"=w1336, "F Values Array"=w1335, "Frekanslar"=w1334, "frekans index"=w1333, "AD F/P Array"=w1330, "10R F/P Array"=w1329, "1R F/P Array"=w1331, "Wagner F/P Array"=w1328, "Kelvin F/P Array"=w1332, "Direnc 1 - Direnc 2"=w1327) -> ("output ad f/p"=w1326:dbl[][], "output 10r f/p"=w1325:dbl[][], "output 1r f/p"=w1324:dbl[][], "output w f/p"=w1323:dbl[][], "output k f/p"=w1322:dbl[][])  [unwired: 5 in]
                                n481 = local write "AD F/P Array"(w1326) -> ()
                                n482 = local write "10R F/P Array"(w1325) -> ()
                                n483 = local write "1R F/P Array"(w1324) -> ()
                                n484 = local write "Wagner F/P Array"(w1323) -> ()
                                n485 = local write "Kelvin F/P Array"(w1322) -> ()
                              }
                            }
                          }
                          frame #1 {
                            n486 = Wait (ms)(milliseconds to wait=u32 150) -> ()  [unwired: 1 out]
                          }
                          frame #2 {
                            n487 = local read "F Values Array"() -> (w1342:dbl[][])
                            n488 = local read "control hz array"() -> (w1341:dbl[][])
                            n489 = local read "extra default values"() -> (w1340:dbl[][])
                            n490 = local read "Frekanslar"() -> (w1344:dbl[])
                            n491 = Build Array(w1344) -> (w1339:dbl[][])
                            n492 = Bundle By Name(cluster="Cluster", "F Values Array"=w1342, "control hz array"=w1341, "extra default values"=w1340, "Frekanslar"=w1339) -> (w1338:T2)
                            n493 = local write "Cluster"(w1338) -> ()
                          }
                          frame #3 {
                            n494 = Wait (ms)(milliseconds to wait=u32 150) -> ()  [unwired: 1 out]
                          }
                          frame #4 {
                            n495 = local read "AD F/P Array"() -> (w1351:dbl[][])
                            n496 = local read "10R F/P Array"() -> (w1350:dbl[][])
                            n497 = local read "1R F/P Array"() -> (w1349:dbl[][])
                            n498 = local read "Wagner F/P Array"() -> (w1348:dbl[][])
                            n499 = local read "Kelvin F/P Array"() -> (w1347:dbl[][])
                            n500 = Bundle By Name(cluster="Cluster 2", "AD F/P Array"=w1351, "10R F/P Array"=w1350, "1R F/P Array"=w1349, "Wagner F/P Array"=w1348, "Kelvin F/P Array"=w1347) -> (w1346:T1)
                            n501 = local write "Cluster 2"(w1346) -> ()
                          }
                        }
                        n502 = flat-sequence {
                          frame #0 {
                            n503 = local read "Frekanslar"() -> (w1274:dbl[])
                            n504 = local read "frekans index"() -> (w1273:dbl)
                            n505 = property on="Default Values Listbox" class="LstBox (strict)"() -> ("Item Names"=w1271:string[])  [unwired: 2 in, 2 out]
                            n506 = Fract/Exp String To Number(string=w1271) -> (number=w1270:dbl[])  [unwired: 3 in, 1 out]
                            n507 = Index Array(array=w1274, index=w1273) -> (element=w1272:dbl)
                            n508 = Search 1D Array(1D array=w1270, element=w1272, start index (0)=0) -> (index of element=w1268:i32)
